vi "Draw Waveform.vi"(8 "Error":errorcluster, 9 "Ref":refnum<vi>, 10 "Data":T2 caption="Data In", 11 "Display State":T1={"Measure ?"=[], "Direction"=[], "Loop ?"={"Start"=0, "Finish"=0}, "Storage Location"=[], "Show Current Location"=FALSE, "Current Location"=0, "Show y=0"=FALSE, "Program"=[], "Index"=0, "Average During Loop ?"=FALSE, "# of Loops"=1, "Loop Control"={0, 2}, "Units"="", "Digits"=0, "Significant Figures (F) or DP (T)"=FALSE, "Rate Mode"=FALSE, "Current Y value"=0.0, "Initial Value"=0.0, "Rate Unit"=""} caption="State" {"# of Loops" min=1 step=1; "Index" min=0 step=1; "Program"."Step" min=0.001 max=80.0 step=0.001 format="%.2f"; "Program"."Target" format="%.2f"}) -> (0 "Error Out":errorcluster, 3 "Display State Out":T1={"Measure ?"=[], "Direction"=[], "Loop ?"={"Start"=0, "Finish"=0}, "Storage Location"=[], "Show Current Location"=FALSE, "Current Location"=0, "Show y=0"=FALSE, "Program"=[], "Index"=0, "Average During Loop ?"=FALSE, "# of Loops"=1, "Loop Control"={0, 2}, "Units"="", "Digits"=0, "Significant Figures (F) or DP (T)"=FALSE, "Rate Mode"=FALSE, "Current Y value"=0.0, "Initial Value"=0.0, "Rate Unit"=""} caption="State" {"# of Loops" min=1 step=1; "Index" min=0 step=1; "Program"."Step" min=0.001 max=80.0 step=0.001 format="%.2f"; "Program"."Target" format="%.2f"})   [LabVIEW 2012, in "Multi Segment Waveform.xctl"]
doc: "Draws the preview plot based on the current XControl state"
uses:
  Multi Segment Waveform.xctl
  Data.ctl
  State.ctl
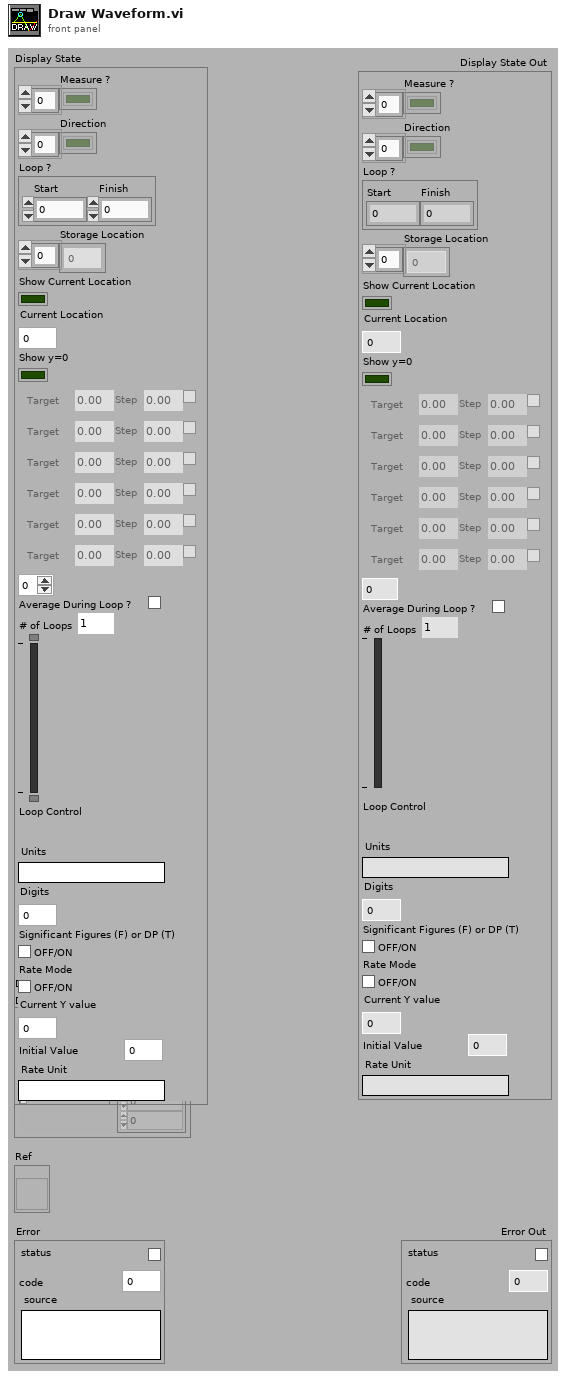
[diagram p1: front panel]
types:
  T1 = typedef "Multi Segment Waveform.xctl/State.ctl" = cluster{"Measure ?":bool[], "Direction":bool[], "Loop ?":cluster{"Start":i32, "Finish":i32}, "Storage Location":i32[], "Show Current Location":bool, "Current Location":i32, "Show y=0":bool, "Program":cluster{"Target":dbl, "Step":dbl, "Measure ?":bool}[], "Index":i32, "Average During Loop ?":bool, "# of Loops":u32, "Loop Control":cluster{i32, i32}, "Units":string, "Digits":i32, "Significant Figures (F) or DP (T)":bool, "Rate Mode":bool, "Current Y value":dbl, "Initial Value":dbl, "Rate Unit":string}
  T2 = typedef "Multi Segment Waveform.xctl/Data.ctl" = waveform(dbl)
  T3 = cluster{"Target":dbl, "Step":dbl, "Measure ?":bool}[]
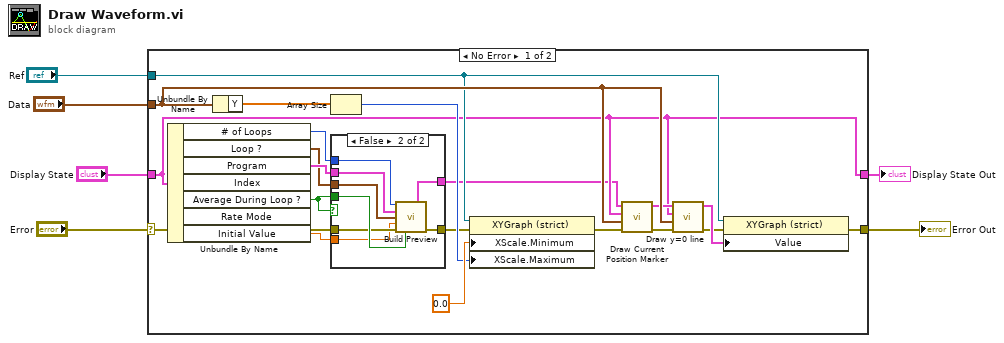
[diagram p0: block diagram]
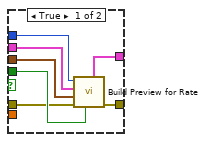
[diagram p2: hidden frame]
diagram:
  n1 = case shown="No Error" "Error" {
    selector: "Error" -> [w10 w43]
    tunnel: "Data" -> [w25 _]
    tunnel: "Display State" -> [w15 w42]
    tunnel: "Ref" -> [w19 _]
    tunnel: [w16 w43] -> w3
    tunnel: [w15 w42] -> w1
    frame No Error {
      n2 = Unbundle By Name(w15) -> ("# of Loops"=w13:u32, "Loop ?"=w12:cluster{"Start":i32, "Finish":i32}, "Program"=w14:T3, "Average During Loop ?"=w8:bool, "Initial Value"=w7:dbl)  [unwired: 2 out]
      n3 = Unbundle By Name(w25) -> ("Y"=w26:dbl[])
      n4 = Array Size(array=w26) -> (size(s)=w21:i32)
      n5 = case shown="False" w8 {
        tunnel: w14 -> [w33 w41]
        tunnel: w13 -> [w32 w40]
        tunnel: w12 -> [w31 w39]
        tunnel: [w30 w38] -> w11
        tunnel: w8 -> [w29 w37]
        tunnel: w10 -> [w28 w36]
        tunnel: [w27 w35] -> w9
        tunnel: w7 -> [_ w34]
        frame True {
          n6 = call "Build Preview for Rate.vi"("Average During Loop ?"=w29, "error in (no error)"=w28, "Loop ?"=w31, "Program"=w33, "# Of Loops"=w32) -> ("error out"=w27:errorcluster, "Plots Out"=w30:cluster{dbl[], dbl[]}[])  [unwired: 5 out]
        }
        frame False {
          n7 = call "Build Preview.vi"("# Of Loops"=w40, "Program"=w41, "Loop ?"=w39, "Initial Value"=w34, "error in (no error)"=w36, "Average During Loop ?"=w37) -> ("Plots Out"=w38:cluster{dbl[], dbl[]}[], "error out"=w35:errorcluster)  [unwired: 3 in, 5 out]
        }
      }
      n8 = property on="Property Node" class="XYGraph (strict)"(reference=w19, error in=w9, "XScale.Minimum"=0.0 ("X Scale.Range:Minimum"), "XScale.Maximum"=w21) -> (error out=w18:errorcluster)  [unwired: 1 out]
      n9 = call "Draw Current Position Marker.vi"("Error"=w18, "Waveform"=w25, "State"=w15, "Plots"=w11) -> ("Error Out"=w24:errorcluster, "Plots Out"=w20:cluster{"X":dbl[], "Y":dbl[]}[])  [unwired: 6 out]
      n10 = call "Draw y=0 line.vi"("Error"=w24, "Waveform"=w25, "State"=w15, "Plots"=w20) -> ("Error Out"=w17:errorcluster, "Plots Out"=w22:cluster{"X":dbl[], "Y":dbl[]}[])  [unwired: 6 out]
      n11 = property class="XYGraph (strict)"(reference=w19, error in=w17, "Value"=w22) -> (error out=w16:errorcluster)  [unwired: 1 out]
    }
    frame Error {
    }
  }
  "Display State Out" <- w1
  "Error Out" <- w3
